vi "Cmd Set Command Properties (C).vi"(4 "error in (no error)":errorcluster, 5 "command properties":T1, 7 "command reference":T2) -> (0 "error out":errorcluster, 3 "command reference out":T2)   [LabVIEW 2012, in "NI_Database_API_64.lvlib"]
doc: "Sets properties on the object as determined by the inputs. Wire data to the reference and properties inputs to determine the polymorphic instance to use or manually select the instance."
uses:
  NI_Database_API_64.lvlib
  Cmd ObjectReference.ctl
  Cmd Properties.ctl
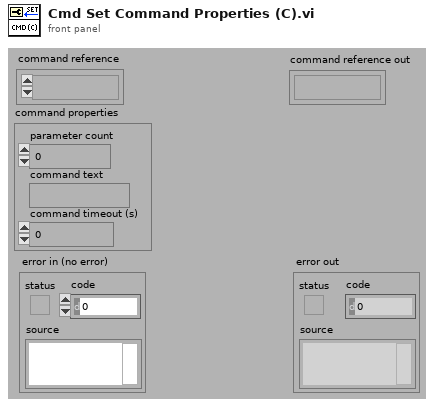
[diagram p1: front panel]
types:
  T1 = typedef "NI_Database_API_64.lvlib/Cmd Properties.ctl" = cluster{"parameter count":i32, "command text":string, "command timeout (s)":i32}
  T2 = typedef "NI_Database_API_64.lvlib/Cmd ObjectReference.ctl" = refnum<k1>
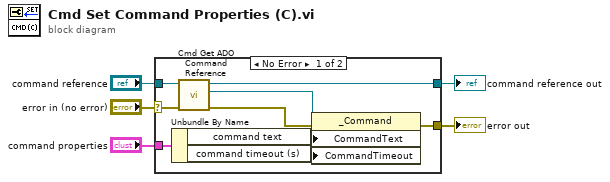
[diagram p0: block diagram]
diagram:
  n1 = case shown="No Error" "error in (no error)" {
    selector: "error in (no error)" -> [w6 w16]
    tunnel: "command reference" -> [w12 w15]
    tunnel: [w11 w15] -> w4
    tunnel: "command properties" -> [w10 _]
    tunnel: [w7 w16] -> w2
    frame No Error {
      n2 = Unbundle By Name(w10) -> ("command text"=w9:string, "command timeout (s)"=w8:i32)
      n3 = call "Cmd Get ADO Command Reference.vi"("error in (no error)"=w6, "command reference"=w12) -> ("error out"=w13:errorcluster, "ADODB._Command"=w14:refnum<k7>, "command reference out"=w11:T2)  [unwired: 3 in]
      n4 = property class="_Command"(reference=w14, error in=w13, "CommandText"=w9, "CommandTimeout"=w8) -> (error out=w7:errorcluster)  [unwired: 1 out]
    }
    frame Error {
    }
  }
  "command reference out" <- w4
  "error out" <- w2
